vi "Module Init.vi"(8 "error in (no error)":errorcluster, 11 "Historian Charting Manager in":refnum<class "Historian Charting Manager.lvclass">) -> (0 "error out":errorcluster, 3 "Historian Charting Manager out":refnum<class "Historian Charting Manager.lvclass">)   [LabVIEW 2020, in "VolatusGUI.lvlib" / "Historian Charting Manager.lvclass"]
uses:
  Historian Charting Manager.lvclass
  Historian Charting Manager.lvclass/Historian Charting Manager.ctl
  Volatus/Module/Module.lvclass
  C:/dev/lv20CE/relink/lv-volatus/Volatus/Module/Module.lvclass
  C:/dev/lv20CE/relink/lv-volatus/VolatusHistorian/Historian Charting Manager/Historian Charting Manager.lvclass
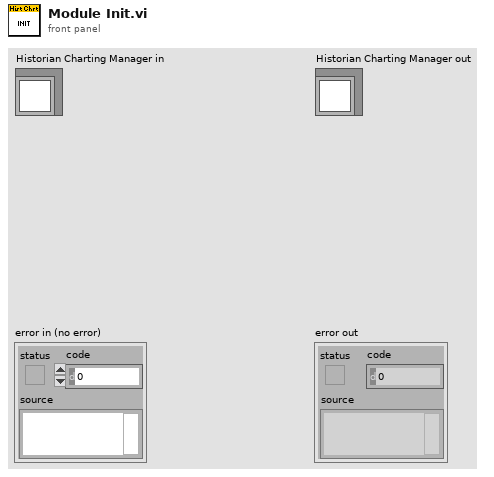
[diagram p1: front panel]
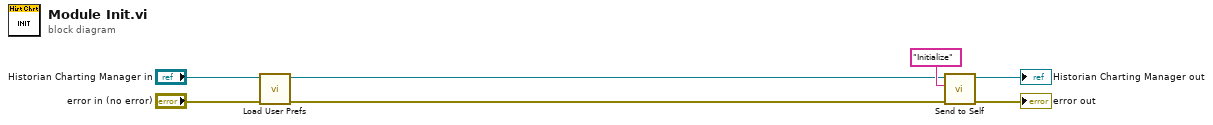
[diagram p0: block diagram]
diagram:
  n1 = call "Load User Prefs.vi"("error in (no error)"="error in (no error)", "Historian Charting Manager in"="Historian Charting Manager in") -> ("error out"=w3:errorcluster, "Historian Charting Manager out"=w1:refnum<class "Historian Charting Manager.lvclass">)  [unwired: 8 in]
  n2 = call "Send to Self.vi"("error in (no error)"=w3, "Message ID"="Initialize", "Module in"=w1) -> ("error out"=→"error out":errorcluster, "Module in"=→"Historian Charting Manager out":refnum<class "Historian Charting Manager.lvclass">)  [unwired: 7 in]
